vi "LbcbConversionLabels.vi"(10 "LbcbConversionType":T2, 11 "LBCB Number":T1) -> (2 "Conversion Label":string)   [LabVIEW 2013]
uses:
  LbcbConversionTypes.ctl
  Data Access Objects/Metadata/LBCB Number.ctl
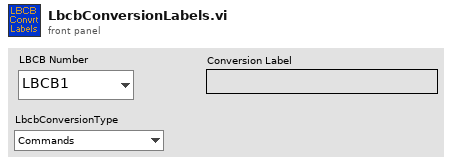
[diagram p1: front panel]
types:
  T1 = typedef "LBCB Number.ctl" = enum16{"LBCB1", "LBCB2"}
  T2 = typedef "LbcbConversionTypes.ctl" = enum16{"Commands", "Readings", "Offsets"}
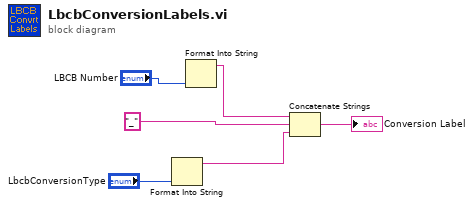
[diagram p0: block diagram]
diagram:
  n1 = Format Into String("LbcbConversionType") -> (resulting string=w2:string)  [unwired: 3 in, 1 out]
  n2 = Format Into String("LBCB Number") -> (resulting string=w5:string)  [unwired: 3 in, 1 out]
  n3 = Concatenate Strings(w5, "_" ("string"), w2) -> (→"Conversion Label":string)
